vi "CRYGet Button State Calibration.vi"(10 "Signal Type Name":string, 11 "Input/Output":bool) -> (0 "Mouth Sim":bool, 1 "Mic or MouseSim State":T1(ring), 2 "Exist":bool, 3 "State":T1(ring), 4 "Mouth Sim Number":i32)   [LabVIEW 2013]
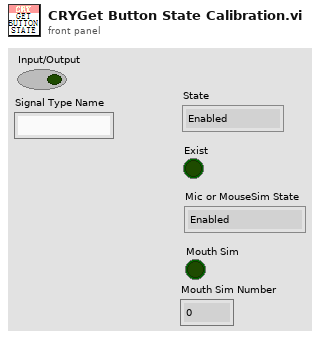
[diagram p1: front panel]
types:
  T1 = enum8{"Enabled", "Disabled", "Disabled and Grayed Out"}
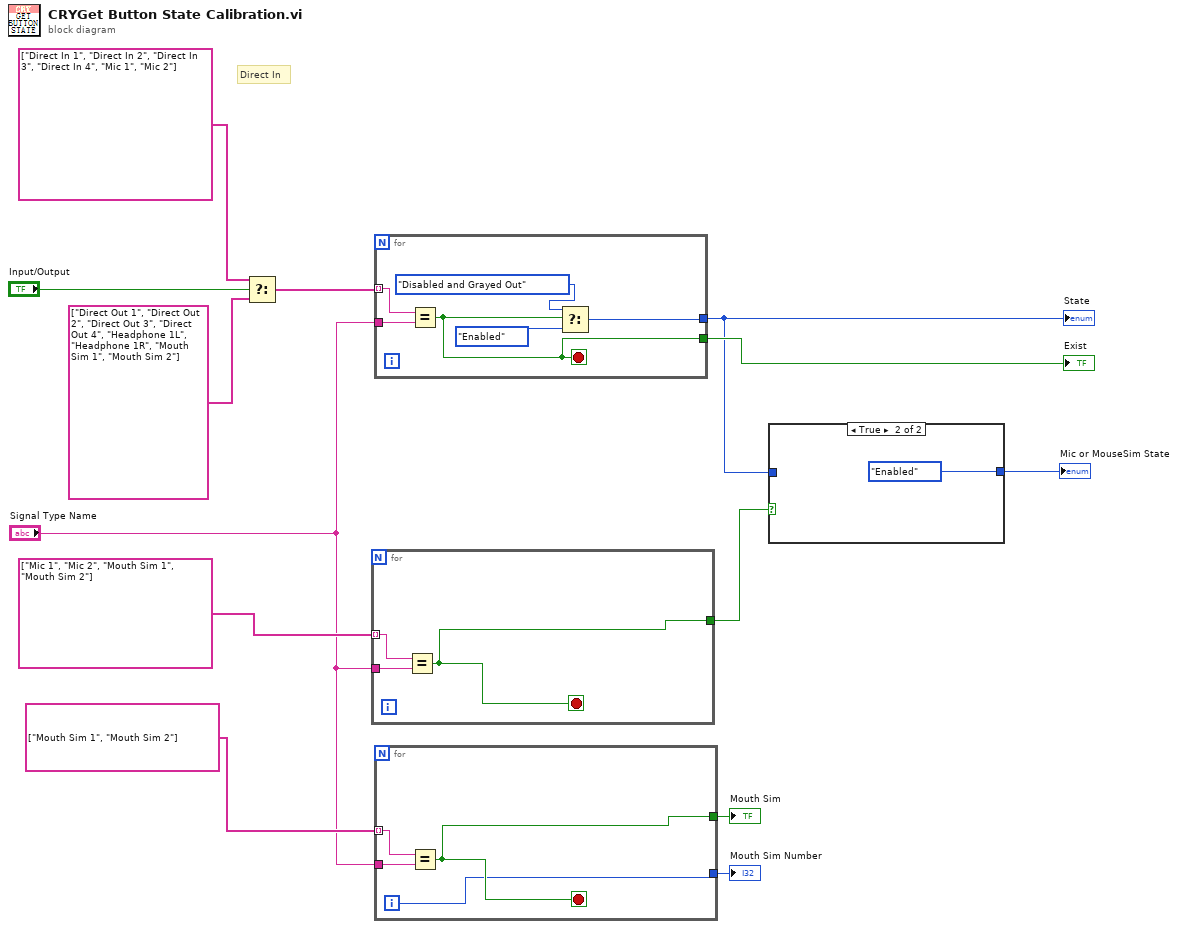
[diagram p0: block diagram]
diagram:
  # "Direct In"
  n1 = Select(t=string[] ["Direct In 1", "Direct In 2", "Direct In 3", "Direct In 4", "Mic 1", "Mic 2"], s="Input/Output", f=string[] ["Direct Out 1", "Direct Out 2", "Direct Out 3", "Direct Out 4", "Headphone 1L", "Headphone 1R", "Mouth Sim 1", "Mouth Sim 2"]) -> (s? t:f=w10:string[])
  n2 = for {
    tunnel: string[] ["Mic 1", "Mic 2", "Mouth Sim 1", "Mouth Sim 2"] -> [w16] mode=indexing
    tunnel: [w14] -> w7
    tunnel: "Signal Type Name" -> [w15]
    stop <- w14 stop-if-true
    n3 = Equal?(x=w16, y=w15) -> (x = y?=w14:bool)
  }
  n4 = for {
    tunnel: w10 -> [w18] mode=indexing
    tunnel: "Signal Type Name" -> [w17]
    tunnel: [w20] -> w6
    tunnel: [w19] -> w8
    stop <- w19 stop-if-true
    n5 = Equal?(x=w18, y=w17) -> (x = y?=w19:bool)
    n6 = Select(t=T1."Disabled and Grayed Out" ("Disabled"), s=w19, f=T1."Enabled") -> (s? t:f=w20:T1)
  }
  "State" <- w6
  "Exist" <- w8
  n7 = for {
    tunnel: string[] ["Mouth Sim 1", "Mouth Sim 2"] -> [w24] mode=indexing
    tunnel: [w25] -> w2
    tunnel: "Signal Type Name" -> [w26]
    tunnel: [w23] -> w1
    i -> [w23]
    stop <- w25 stop-if-true
    n8 = Equal?(x=w24, y=w26) -> (x = y?=w25:bool)
  }
  "Mouth Sim" <- w2
  "Mouth Sim Number" <- w1
  n9 = case shown="True" w7 {
    tunnel: w6 -> [w27 _]
    tunnel: [w27 T1."Enabled" ("f")] -> w5
    frame False {
    }
    frame True {
    }
  }
  "Mic or MouseSim State" <- w5
